vi "AdjustTable.vi"(8 "error in (no error)":errorcluster, 10 "AllVirtualTypeData":T1={"Search Name"="", "Start X"=0.0, "Increase X"=0.0, "X Step"=1, "Start Y"=0.0, "Increase Y"=0.0, "Y Step"=1, "Sensor"=0} {"Y Step" min=1 step=1; "X Step" min=1 step=1}) -> (0 "error out":errorcluster, 1 "VirtualYArray":dbl[](array[numeric]), 2 "VirtualXArray":dbl[](array[numeric]), 5 "Sensor":i32)   [LabVIEW 2014, in "VirtualOrigin.lvclass"]
uses:
  VirtualOrigin.lvclass
  Control/AllVirtualTypeData.ctl
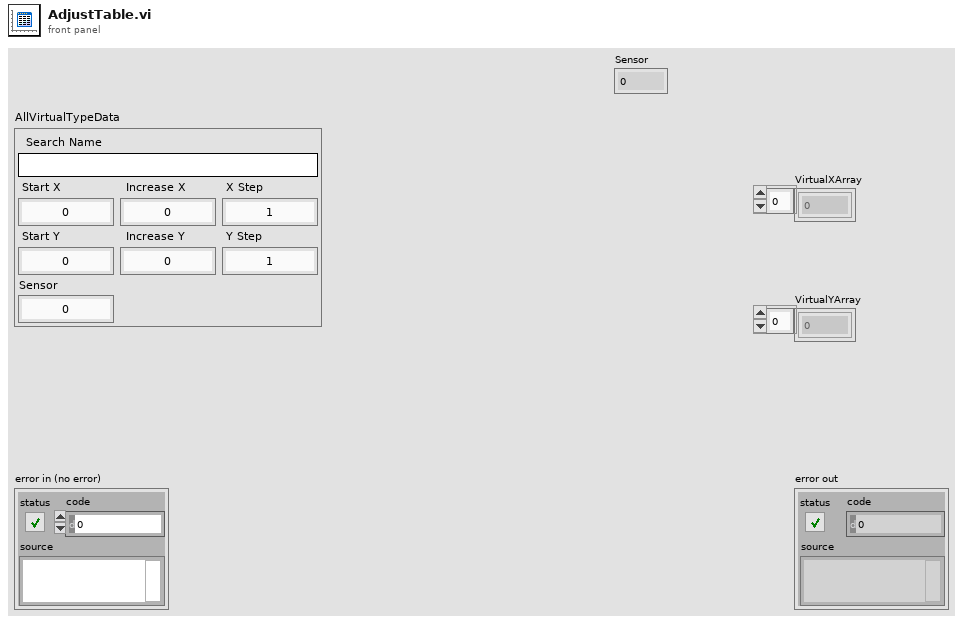
[diagram p1: front panel]
types:
  T1 = typedef "VirtualOrigin.lvclass/AllVirtualTypeData.ctl" = cluster{"Search Name":string, "Start X":dbl, "Increase X":dbl, "X Step":i32, "Start Y":dbl, "Increase Y":dbl, "Y Step":i32, "Sensor":i32}
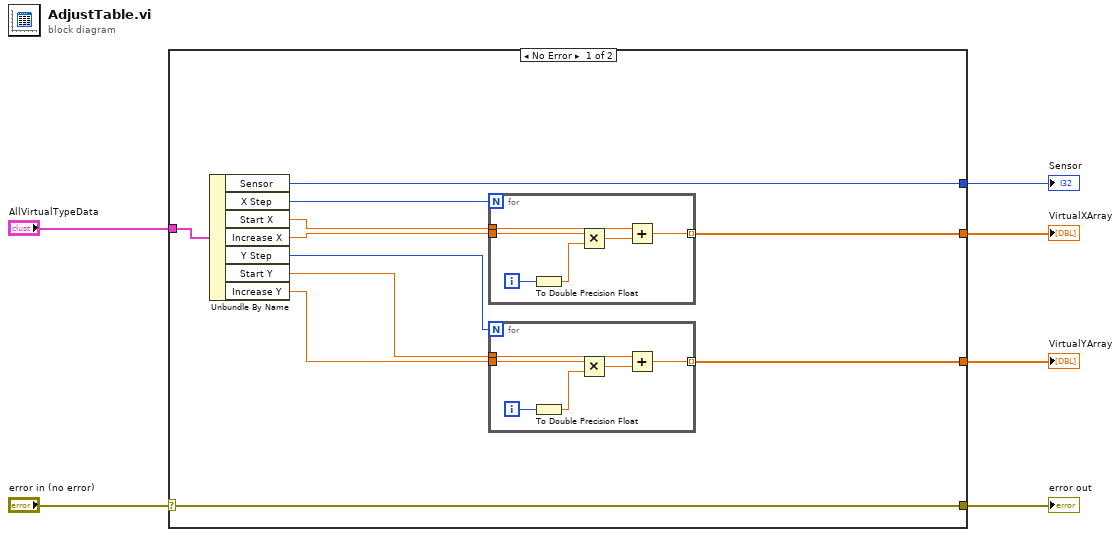
[diagram p0: block diagram]
diagram:
  n1 = case shown="No Error" "error in (no error)" {
    selector: "error in (no error)" -> [w17 w30]
    tunnel: [w17 w30] -> w5
    tunnel: "AllVirtualTypeData" -> [w10 _]
    tunnel: [w9 _] -> w3
    tunnel: [w8 _] -> w2
    tunnel: [w7 _] -> w1
    frame No Error {
      n2 = Unbundle By Name(w10) -> ("Sensor"=w9:i32, "X Step"=w11:i32, "Start X"=w15:dbl, "Increase X"=w16:dbl, "Y Step"=w12:i32, "Start Y"=w13:dbl, "Increase Y"=w14:dbl)
      n3 = for {
        N: w11 -> [_]
        tunnel: w15 -> [w29]
        tunnel: [w26] -> w8 mode=indexing
        tunnel: w16 -> [w25]
        i -> [w28]
        n4 = To Double Precision Float(number=w28) -> (double precision float=w27:dbl)
        n5 = Multiply(x=w25, y=w27) -> (x*y=w24:dbl)
        n6 = Add(x=w29, y=w24) -> (x+y=w26:dbl)
      }
      n7 = for {
        N: w12 -> [_]
        tunnel: w13 -> [w23]
        tunnel: [w20] -> w7 mode=indexing
        tunnel: w14 -> [w19]
        i -> [w22]
        n8 = To Double Precision Float(number=w22) -> (double precision float=w21:dbl)
        n9 = Multiply(x=w19, y=w21) -> (x*y=w18:dbl)
        n10 = Add(x=w23, y=w18) -> (x+y=w20:dbl)
      }
    }
    frame Error {
    }
  }
  "error out" <- w5
  "Sensor" <- w3
  "VirtualXArray" <- w2
  "VirtualYArray" <- w1
